vi "Set Configuration Parameter - Boolean.vi"(7 "Section":string, 8 "error in (no error)":errorcluster, 9 "Value":bool, 10 "Key":string, 11 "Ethernet in":refnum<class "ENET_BS1201.lvclass">) -> (0 "error out":errorcluster, 3 "Ethernet out":refnum<class "ENET_BS1201.lvclass">)   [LabVIEW 2021, in "BS120x Driver.lvlib" / "ENET_BS1201.lvclass"]
uses:
  ENET_BS1201.lvclass
  C:/Users/Public/Documents/Projects/7100-00109 SW BS1201 LV Driver/trunk/source/ENET_BS120x/ENET_BS120x.lvclass
  ENET_BS1201.lvclass/ENET_BS1201.ctl
  ENET_BS120x/ENET_BS120x.lvclass
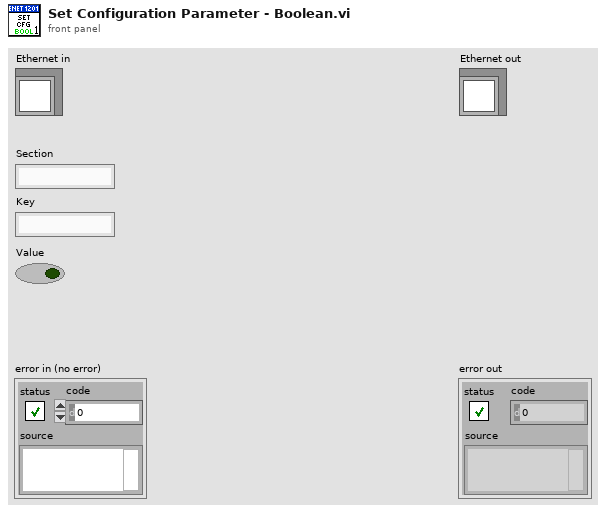
[diagram p1: front panel]
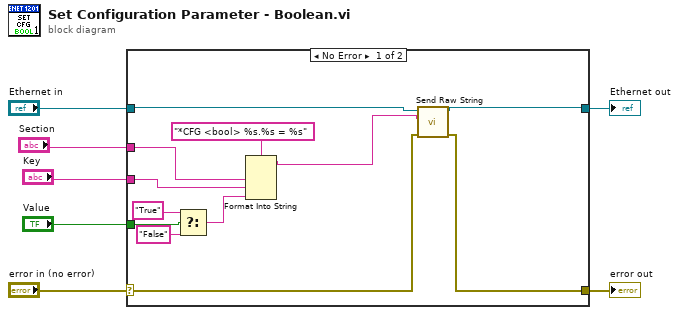
[diagram p0: block diagram]
diagram:
  n1 = case shown="No Error" "error in (no error)" {
    selector: "error in (no error)" -> [w9 w21]
    tunnel: [w8 w21] -> w6
    tunnel: [w10 w20] -> w4
    tunnel: "Ethernet in" -> [w12 w20]
    tunnel: "Section" -> [w18 _]
    tunnel: "Key" -> [w17 _]
    tunnel: "Value" -> [w16 _]
    frame No Error {
      n2 = Select(t="True" ("format string"), s=w16, f="False" ("format string")) -> (s? t:f=w13:string)
      n3 = Format Into String(format string="*CFG <bool> %s.%s = %s", w18, w17, w13) -> (resulting string=w11:string)  [unwired: 2 in, 1 out]
      n4 = call "Send Raw String.vi"("error in (no error)"=w9, "String Data"=w11, "ENET in"=w12) -> ("error out"=w8:errorcluster, "ENET out"=w10:refnum<class "ENET_BS1201.lvclass">)  [unwired: 7 in]
    }
    frame Error {
    }
  }
  "error out" <- w6
  "Ethernet out" <- w4
